vi "Pre Launch Init.vi"(11 "CS++DSCMonitor in":refnum<class "CS++DSCMonitor.lvclass">) -> (0 "error out":errorcluster, 3 "CS++DSCMonitor out":refnum<class "CS++DSCMonitor.lvclass">)   [LabVIEW 2014, in "CS++DSCMonitor.lvlib" / "CS++DSCMonitor.lvclass"]
doc: "(<B>Filename</B>: Actor Framework.lvlib:Actor.lvclass:Pre Launch Init.vi)\n\nDefines behavior that occurs after the Launch Actor method is invoked but before the actor's Actor Core method begins running.\n\nThe Pre Launch Init method is guaranteed to finish before the Launch Actor method returns to its caller and before the actor itself receives any messages. Any references that the Pre Launch Init method obtains are guaranteed to have the same lifetime as the actor itself. Any errors that the Pre Launch Init method returns will abort the launch.\n\nBy default, this method does nothing. A descendant class may override it to define behavior."
uses:
  CS++DSCMonitor.lvclass
  <vilib>/ActorFramework/Message Enqueuer/Message Enqueuer.lvclass
  CSPP_Core/Actors/CS++PVMonitor Messages/CS++AEUpdate Msg/CS++AEUpdate Msg.lvclass
  CSPP_Core/Actors/CS++SVMonitor/CS++SVMonitor.lvclass/CS++SVMonitor.ctl
  CS++DSCMonitor.lvclass/CS++DSCMonitor.ctl
  CSPP_Core/Actors/CS++SVMonitor/CS++SVMonitor.lvclass
  CSPP_Core/Actors/CS++PVMonitor Messages/CS++PVUpdate Msg/CS++PVUpdate Msg.lvclass
  <vilib>/lvdsc/NI_DSC.lvlib
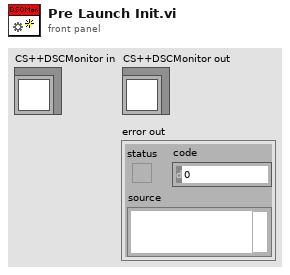
[diagram p1: front panel]
types:
  T1 = cluster{"AE URL":string, "Observers":cluster{"Enqueuer":refnum<class "Message Enqueuer.lvclass">, "CS++AEUpdate Msg":refnum<class "CS++AEUpdate Msg.lvclass">}[]}[]
  T2 = cluster{"Stop":refnum<user-event>, "PV Connections":refnum<user-event>}
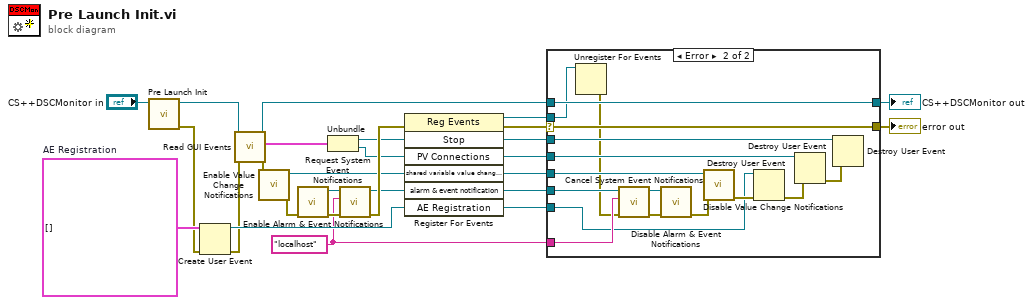
[diagram p0: block diagram]
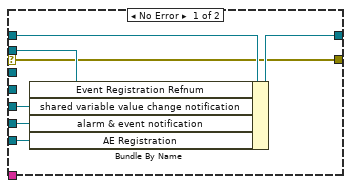
[diagram p2: hidden frame]
diagram:
  w1 = "localhost" ("server (localhost)")
  w21 = T1 []  # AE Registration
  n1 = call-parent "Pre Launch Init.vi"("CS++SVMonitor in"="CS++DSCMonitor in") -> ("error out"=w20:errorcluster, "CS++SVMonitor out"=w12:refnum<class "CS++DSCMonitor.lvclass">)  [unwired: 9 in]
  n2 = Create User Event(user event datatype=w21, error in=w20) -> (user event=w10:refnum<user-event>, error out=w6:errorcluster)
  n3 = call "Read GUI Events.vi"("error in (no error)"=w6, "CS++SVMonitor in"=w12) -> ("error out"=w14:errorcluster, "GUI Events"=w13:T2, "CS++SVMonitor out"=w11:refnum<class "CS++DSCMonitor.lvclass">)  [unwired: 7 in]
  n4 = call <vilib>:"Enable Value Change Notifications.vi"("error in (no error)"=w14) -> ("error out"=w15:errorcluster, "shared variable value change notification"=w8:refnum<user-event>)  [unwired: 9 out]
  n5 = call <vilib>:"Enable Alarm & Event Notifications.vi"("error in (no error)"=w15) -> ("error out"=w17:errorcluster, "alarm & event notification"=w16:refnum<user-event>)  [unwired: 9 out]
  n6 = Unbundle(w13) -> ("Stop"=w3:refnum<user-event>, "PV Connections"=w2:refnum<user-event>)
  n7 = call <vilib>:"Request System Event Notifications.vi"("error in (no error)"=w17, "server (localhost)"=w1, "notification refnum"=w16) -> ("error out"=w18:errorcluster, "alarm & event notification"=w9:refnum<user-event>)  [unwired: 6 in, 1 out]
  n8 = register-events(error in=w18, w3, w2, w8, w9, w10) -> (reference out=w7:refnum<event-registration>, error out=w5:errorcluster)  [unwired: 1 in]
  n9 = case shown="Error" w5 {
    selector: w5 -> [w23 w44]
    tunnel: [w29 w45] -> w19
    tunnel: w11 -> [w28 w45]
    tunnel: w10 -> [w27 w30]
    tunnel: w9 -> [w26 w33]
    tunnel: w8 -> [w25 w35]
    tunnel: w7 -> [w24 w38]
    tunnel: [w23 w44] -> w4
    tunnel: w3 -> [_ w37]
    tunnel: w2 -> [_ w36]
    tunnel: w1 -> [_ w34]
    frame No Error {
      n10 = Bundle By Name(cluster=w28, "Event Registration Refnum"=w24, "shared variable value change notification"=w25, "alarm & event notification"=w26, "AE Registration"=w27) -> (w29:refnum<class "CS++DSCMonitor.lvclass">)
    }
    frame Error {
      n11 = Unregister For Events(event registration refnum=w38) -> (error out=w32:errorcluster)  [unwired: 1 in]
      n12 = call <vilib>:"Cancel System Event Notifications.vi"("error in (no error)"=w32, "server (localhost)"=w34, "notification refnum"=w33) -> ("error out"=w42:errorcluster, "alarm & event notification"=w43:refnum<user-event>)  [unwired: 6 in, 1 out]
      n13 = call <vilib>:"Disable Alarm & Event Notifications.vi"("error in (no error)"=w42, "notification refnum"=w43) -> ("error out"=w31:errorcluster)  [unwired: 9 out]
      n14 = call <vilib>:"Disable Value Change Notifications.vi"("error in (no error)"=w31, "notification refnum"=w35) -> ("error out"=w41:errorcluster)  [unwired: 9 out]
      n15 = Destroy User Event(user event=w30, error in=w41) -> (error out=w40:errorcluster)
      n16 = Destroy User Event(user event=w36, error in=w40) -> (error out=w39:errorcluster)
      n17 = Destroy User Event(user event=w37, error in=w39) -> ()  [unwired: 1 out]
    }
  }
  "error out" <- w4
  "CS++DSCMonitor out" <- w19
